vi "Apply main gui values to calib toolbox.vi"(8 "error in (no error)":errorcluster, 11 "Calibration GUI parameters in":T1) -> (0 "error out":errorcluster)   [LabVIEW 2020]
uses:
  TypeDefs/Calibration GUI parameter refs.ctl
  Global Variables/gl_UI Ctrl Refs.vi
  Typedefs/Objective selector control enum.ctl
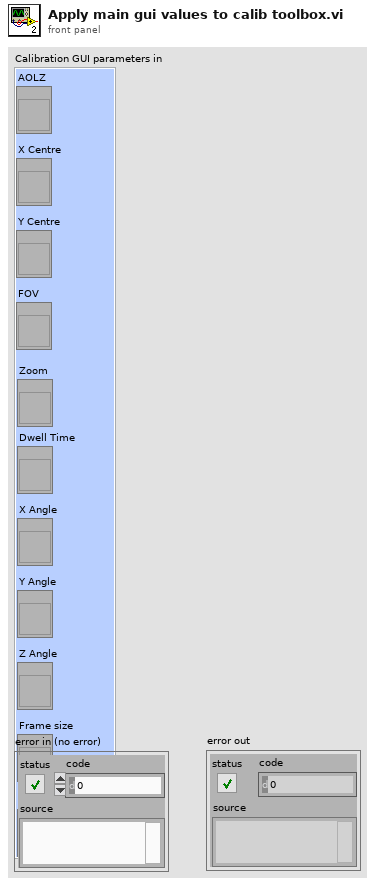
[diagram p1: front panel]
types:
  T1 = typedef "Calibration GUI parameter refs.ctl" = cluster{"AOLZ":refnum<vi>, "X Centre":refnum<vi>, "Y Centre":refnum<vi>, "FOV":refnum<vi>, "Dwell Time":refnum<vi>, "X Angle":refnum<vi>, "Y Angle":refnum<vi>, "Z Angle":refnum<vi>, "Frame size":refnum<vi>, "Current Objective":refnum<vi>, "Zoom":refnum<vi>}
  T2 = typedef "UI ctrl refs cluster.ctl" = cluster{"Top level VI path":path, "Top level VI ref":refnum<vi>, "User menu ref":refnum<k9>, "Sub Panel control":refnum<vi>, "Imaging Param Tab":refnum<vi>, "Occurrence-Start drivers":refnum<k4>, "Occurrence-Speed logging initialised":refnum<k4>, "Occurrence-XYZ stage initialised":refnum<k4>, "Exit button":refnum<vi>, "Status ind":refnum<vi>, "Set as origin":refnum<vi>, "Speed Logging":refnum<vi>, "Time Lapse":refnum<vi>, "Live Imaging":refnum<vi>, "AOL Z Stack":refnum<vi>, "Motor Z Stack":refnum<vi>, "Funct Acq button":refnum<vi>, "Hard Shutter":refnum<vi>, "Virtual Shutter":refnum<vi>, "Laser Power":refnum<vi>, "AOL Mode":refnum<vi>, "Frame Size":refnum<vi>, "Field of View":refnum<vi>, "Dwell Time":refnum<vi>, "Zoom":refnum<vi>, "AOL Z":refnum<vi>, "Objective":refnum<vi>, "Axis":refnum<vi>, "Paths & Names":refnum<vi>, "Experiment folder path (ind.)":refnum<vi>, "Last State (Ind.)":refnum<vi>, "Averages":refnum<vi>, "Angle (degrees)":refnum<vi>, "X centre":refnum<vi>, "Y centre":refnum<vi>, "Plane Mode":refnum<vi>, "# Planes":refnum<vi>, "Z Start":refnum<vi>, "Z Stop":refnum<vi>, "Z Step":refnum<vi>, "PMT 1":refnum<vi>, "PMT 2":refnum<vi>, "Stage XYZ Position":refnum<vi>, "Pockels@Z Start":refnum<vi>, "Pockels@Z Stop":refnum<vi>, "Obtain Z Start":refnum<vi>, "Obtain Z Stop":refnum<vi>, "Live stim.trig.period":refnum<vi>, "Live stim.trig.enable":refnum<vi>, "Movement Correction":refnum<vi>, "Load Reference Image":refnum<vi>, "XY Stage Move":refnum<vi>, "MovCor Cluster":refnum<vi>, "RefDAQParam":refnum<vi>, "Funct. Acq. Pockels Modulation":refnum<vi>, "Ref Laser Power":refnum<vi>, "Enable Video Recording":refnum<vi>, "Video Record-Live Imaging":refnum<vi>, "Video Record-Funct acq":refnum<vi>, "Reference Source":refnum<vi>, "AOL Z-stack Chirps Ready (ind)":refnum<vi>, "Target time between mov.cor. ref triggers (ms)":refnum<vi>, "Funct. Acq. Ref frame save":refnum<vi>, "Tracking button":refnum<vi>, "Show ref plots window":refnum<vi>, "Center freq ind (nm)":refnum<vi>, "Pickup mode (ind)":refnum<vi>, "Logging queue (ind)":refnum<vi>, "Back aperture power (ind.)":refnum<vi>, "Power after objective (ind.)":refnum<vi>, "Switch user":refnum<vi>, "Ls1 Conn. Status":refnum<vi>, "Ls1Tuning Status":refnum<vi>, "Ls1 Faults":refnum<vi>, "Ls1 Connection":refnum<vi>, "Ls1 Mode":refnum<vi>, "Ls1 POWER [mW]":refnum<vi>, "Ls1Shutter":refnum<vi>, "Ls1 Wavelength":refnum<vi>, "Ls1 Note":refnum<vi>, "Ls1 Confirm Wav":refnum<vi>, "Ls1 PreChrp Prism1":refnum<vi>, "Ls1 PreChrp Prism2":refnum<vi>, "Ls1 wav top Ind":refnum<vi>, "Ls1 power top Ind":refnum<vi>, "Ls1 Pump peak Hold":refnum<vi>, "Ls1 Status Ind":refnum<vi>, "Ls1 wav cancel":refnum<vi>, "Experiment Type":refnum<vi>, "Biology Information":refnum<vi>}
  T3 = typedef "Frame Size.ctl" = u16
  T4 = typedef "Plane Mode.ctl" = u16
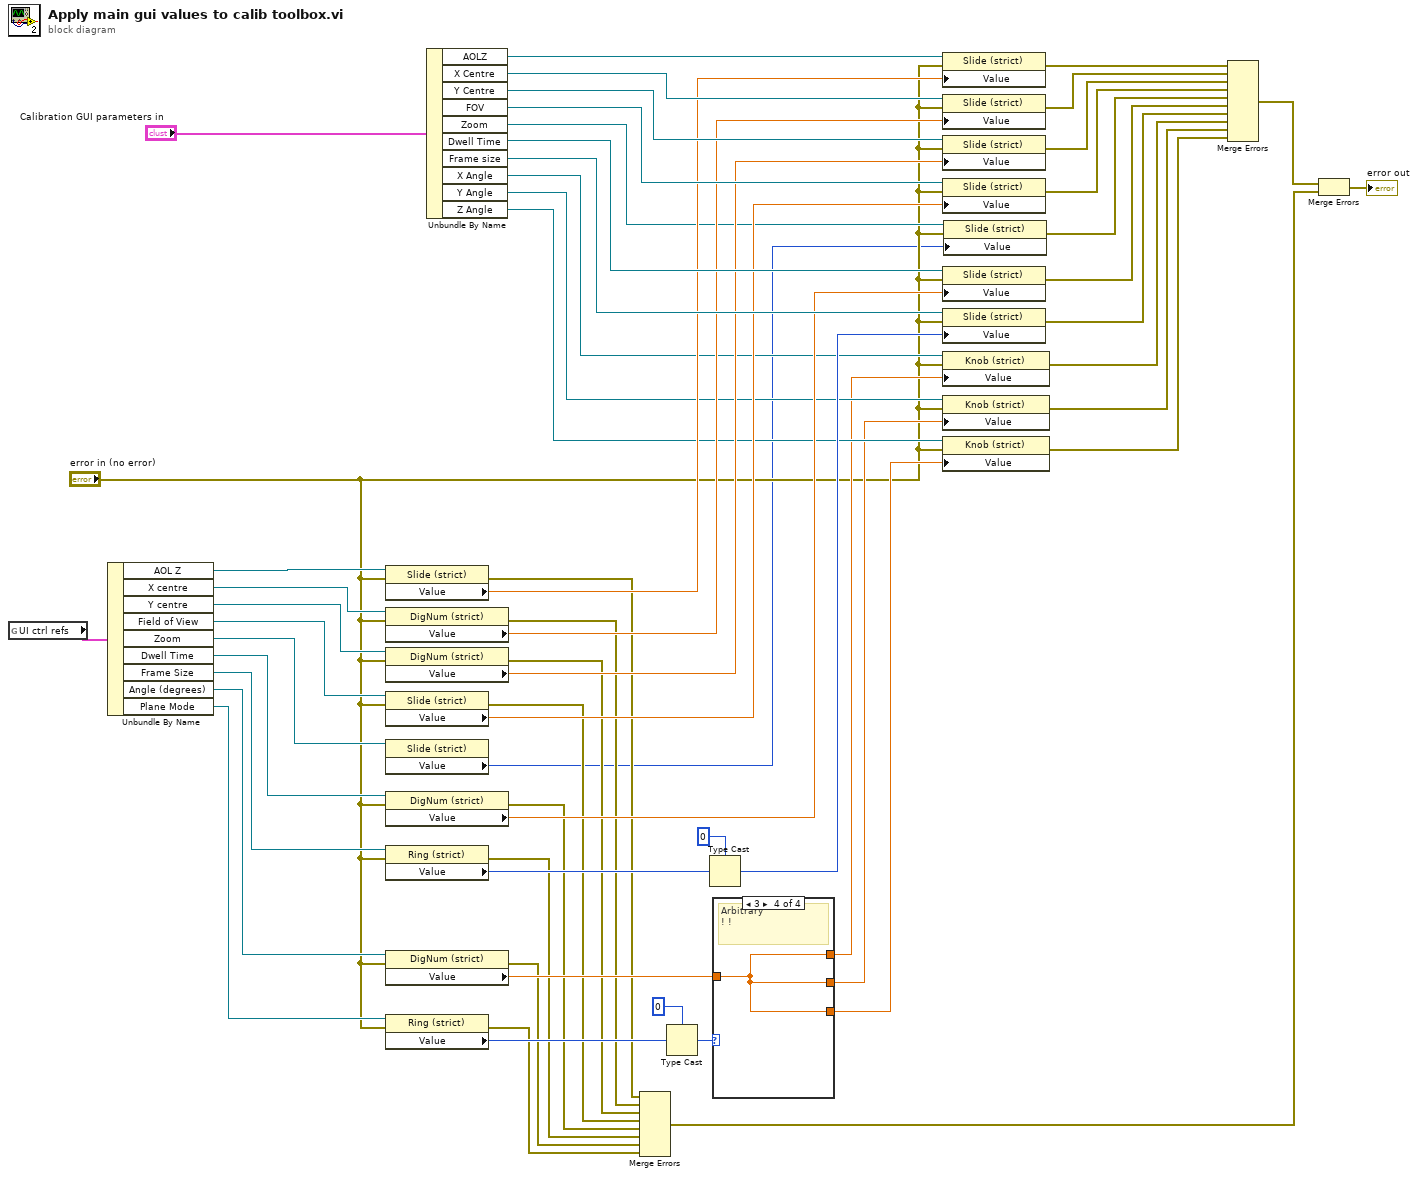
[diagram p0: block diagram]
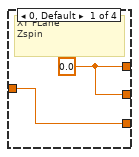
[diagram p2: hidden frame]
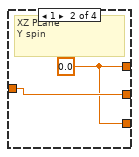
[diagram p3: hidden frame]
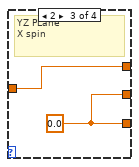
[diagram p4: hidden frame]
diagram:
  n1 = global read "gl_UI Ctrl Refs.vi" "UI ctrl refs"() -> (w59:T2)
  n2 = Unbundle By Name(w59) -> ("AOL Z"=w51:refnum<vi>, "X centre"=w50:refnum<vi>, "Y centre"=w49:refnum<vi>, "Field of View"=w48:refnum<vi>, "Zoom"=w5:refnum<vi>, "Dwell Time"=w47:refnum<vi>, "Frame Size"=w39:refnum<vi>, "Angle (degrees)"=w46:refnum<vi>, "Plane Mode"=w45:refnum<vi>)
  n3 = property class="Slide (strict)"(reference=w51, error in="error in (no error)") -> (error out=w25:errorcluster, "Value"=w44:sgl)  [unwired: 1 out]
  n4 = property class="DigNum (strict)"(reference=w50, error in="error in (no error)") -> (error out=w24:errorcluster, "Value"=w43:dbl)  [unwired: 1 out]
  n5 = property class="DigNum (strict)"(reference=w49, error in="error in (no error)") -> (error out=w23:errorcluster, "Value"=w42:dbl)  [unwired: 1 out]
  n6 = property class="Slide (strict)"(reference=w48, error in="error in (no error)") -> (error out=w22:errorcluster, "Value"=w41:sgl)  [unwired: 1 out]
  n7 = property class="Slide (strict)"(reference=w5) -> ("Value"=w2:i8)  [unwired: 1 in, 2 out]
  n8 = property class="DigNum (strict)"(reference=w47, error in="error in (no error)") -> (error out=w21:errorcluster, "Value"=w40:dbl)  [unwired: 1 out]
  n9 = property class="Ring (strict)"(reference=w39, error in="error in (no error)") -> (error out=w20:errorcluster, "Value"=w37:T3)  [unwired: 1 out]
  n10 = property class="DigNum (strict)"(reference=w46, error in="error in (no error)") -> (error out=w19:errorcluster, "Value"=w32:dbl)  [unwired: 1 out]
  n11 = property class="Ring (strict)"(reference=w45, error in="error in (no error)") -> (error out=w18:errorcluster, "Value"=w34:T4)  [unwired: 1 out]
  n12 = Unbundle By Name("Calibration GUI parameters in") -> ("AOLZ"=w57:refnum<vi>, "X Centre"=w56:refnum<vi>, "Y Centre"=w55:refnum<vi>, "FOV"=w54:refnum<vi>, "Zoom"=w4:refnum<vi>, "Dwell Time"=w53:refnum<vi>, "Frame size"=w52:refnum<vi>, "X Angle"=w31:refnum<vi>, "Y Angle"=w30:refnum<vi>, "Z Angle"=w29:refnum<vi>)
  n13 = Merge Errors(w25, w24, w23, w22, w21, w20, w19, w18) -> (w7:errorcluster)
  n14 = Type Cast(type=u16 0, x=w34) -> (*(type *) &x=w33:u16)
  n15 = Type Cast(type=u16 0 ("Value"), x=w37) -> (*(type *) &x=w36:u16)
  n16 = case shown="3" w33 {
    tunnel: [w60 w62 w65 w66] -> w28
    tunnel: [w60 w63 w64 w66] -> w27
    tunnel: [w61 w62 w64 w66] -> w26
    tunnel: w32 -> [w61 w63 w65 w66]
    frame 0, Default {
      w60 = 0.0
      # "XY PLane\nZspin"
    }
    frame 1 {
      w62 = 0.0
      # "XZ PLane\nY spin"
    }
    frame 2 {
      w64 = 0.0 ("Value")
      # "YZ PLane\nX spin"
    }
    frame 3 {
      # "Arbitrary\n! !"
    }
  }
  n17 = property class="Slide (strict)"(reference=w57, error in="error in (no error)", "Value"=w44) -> (error out=w17:errorcluster)  [unwired: 1 out]
  n18 = property class="Slide (strict)"(reference=w56, error in="error in (no error)", "Value"=w43) -> (error out=w16:errorcluster)  [unwired: 1 out]
  n19 = property class="Slide (strict)"(reference=w55, error in="error in (no error)", "Value"=w42) -> (error out=w15:errorcluster)  [unwired: 1 out]
  n20 = property class="Slide (strict)"(reference=w54, error in="error in (no error)", "Value"=w41) -> (error out=w14:errorcluster)  [unwired: 1 out]
  n21 = property class="Slide (strict)"(reference=w53, error in="error in (no error)", "Value"=w40) -> (error out=w13:errorcluster)  [unwired: 1 out]
  n22 = property class="Slide (strict)"(reference=w52, error in="error in (no error)", "Value"=w36) -> (error out=w12:errorcluster)  [unwired: 1 out]
  n23 = property class="Knob (strict)"(reference=w31, error in="error in (no error)", "Value"=w28) -> (error out=w11:errorcluster)  [unwired: 1 out]
  n24 = property class="Knob (strict)"(reference=w30, error in="error in (no error)", "Value"=w27) -> (error out=w10:errorcluster)  [unwired: 1 out]
  n25 = property class="Knob (strict)"(reference=w29, error in="error in (no error)", "Value"=w26) -> (error out=w9:errorcluster)  [unwired: 1 out]
  n26 = property class="Slide (strict)"(reference=w4, error in="error in (no error)", "Value"=w2) -> (error out=w1:errorcluster)  [unwired: 1 out]
  n27 = Merge Errors(w17, w16, w15, w14, w1, w13, w12, w11, w10, w9) -> (w8:errorcluster)
  n28 = Merge Errors(w8, w7) -> (→"error out":errorcluster)
